vi "APDStageScan.vi"(3 "error in (no error)":errorcluster, 4 "Take Trajectory?":bool, 5 "Scanning parameters":T1) -> (0 "error out":errorcluster, 2 "output array":u32[][](array[numeric]))   [LabVIEW 2015]
uses:
  <vilib>/DAQmx/write.llb/DAQmx Write (Analog 1D Wfm NChan NSamp).vi
  <vilib>/DAQmx/write.llb/DAQmx Write (Digital Bool 1Line 1Point).vi
  <vilib>/DAQmx/read.llb/DAQmx Read (Counter 1D U32 1Chan NSamp).vi
  <vilib>/DAQmx/create/channels.llb/DAQmx Create Channel (CI-Period).vi
  <vilib>/DAQmx/configure/timing.llb/DAQmx Timing (Implicit).vi
  <vilib>/DAQmx/create/channels.llb/DAQmx Create Channel (AO-Voltage-Basic).vi
  <vilib>/DAQmx/create/channels.llb/DAQmx Create Channel (CO-Pulse Generation-Frequency).vi
  <vilib>/DAQmx/configure/timing.llb/DAQmx Timing (Sample Clock).vi
  <vilib>/DAQmx/miscellaneous.llb/DAQmx Fill In Error Info.vi
  <vilib>/DAQmx/create/channels.llb/DAQmx Create Channel (DO-Digital Output).vi
  <resource>/objmgr/daqmx.rc
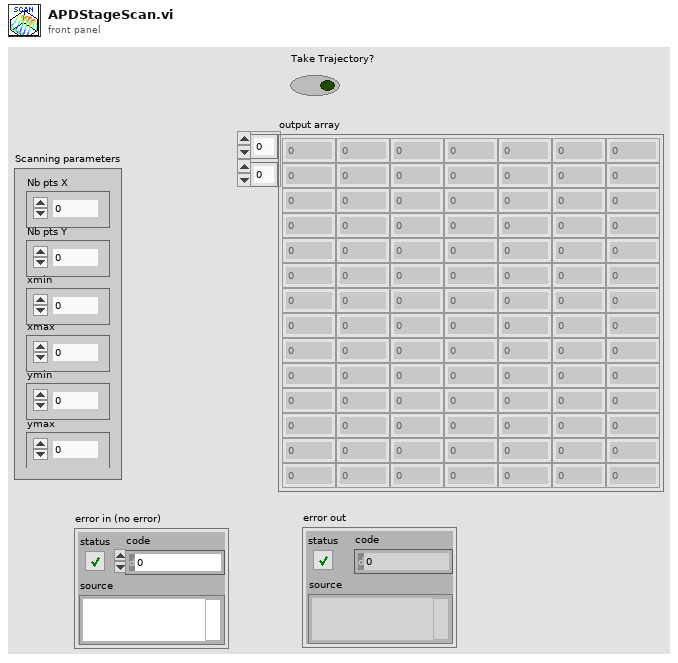
[diagram p1: front panel]
types:
  T1 = cluster{"Nb pts X":u32, "Nb pts Y":u32, "xmin":dbl, "xmax":dbl, "ymin":dbl, "ymax":dbl}
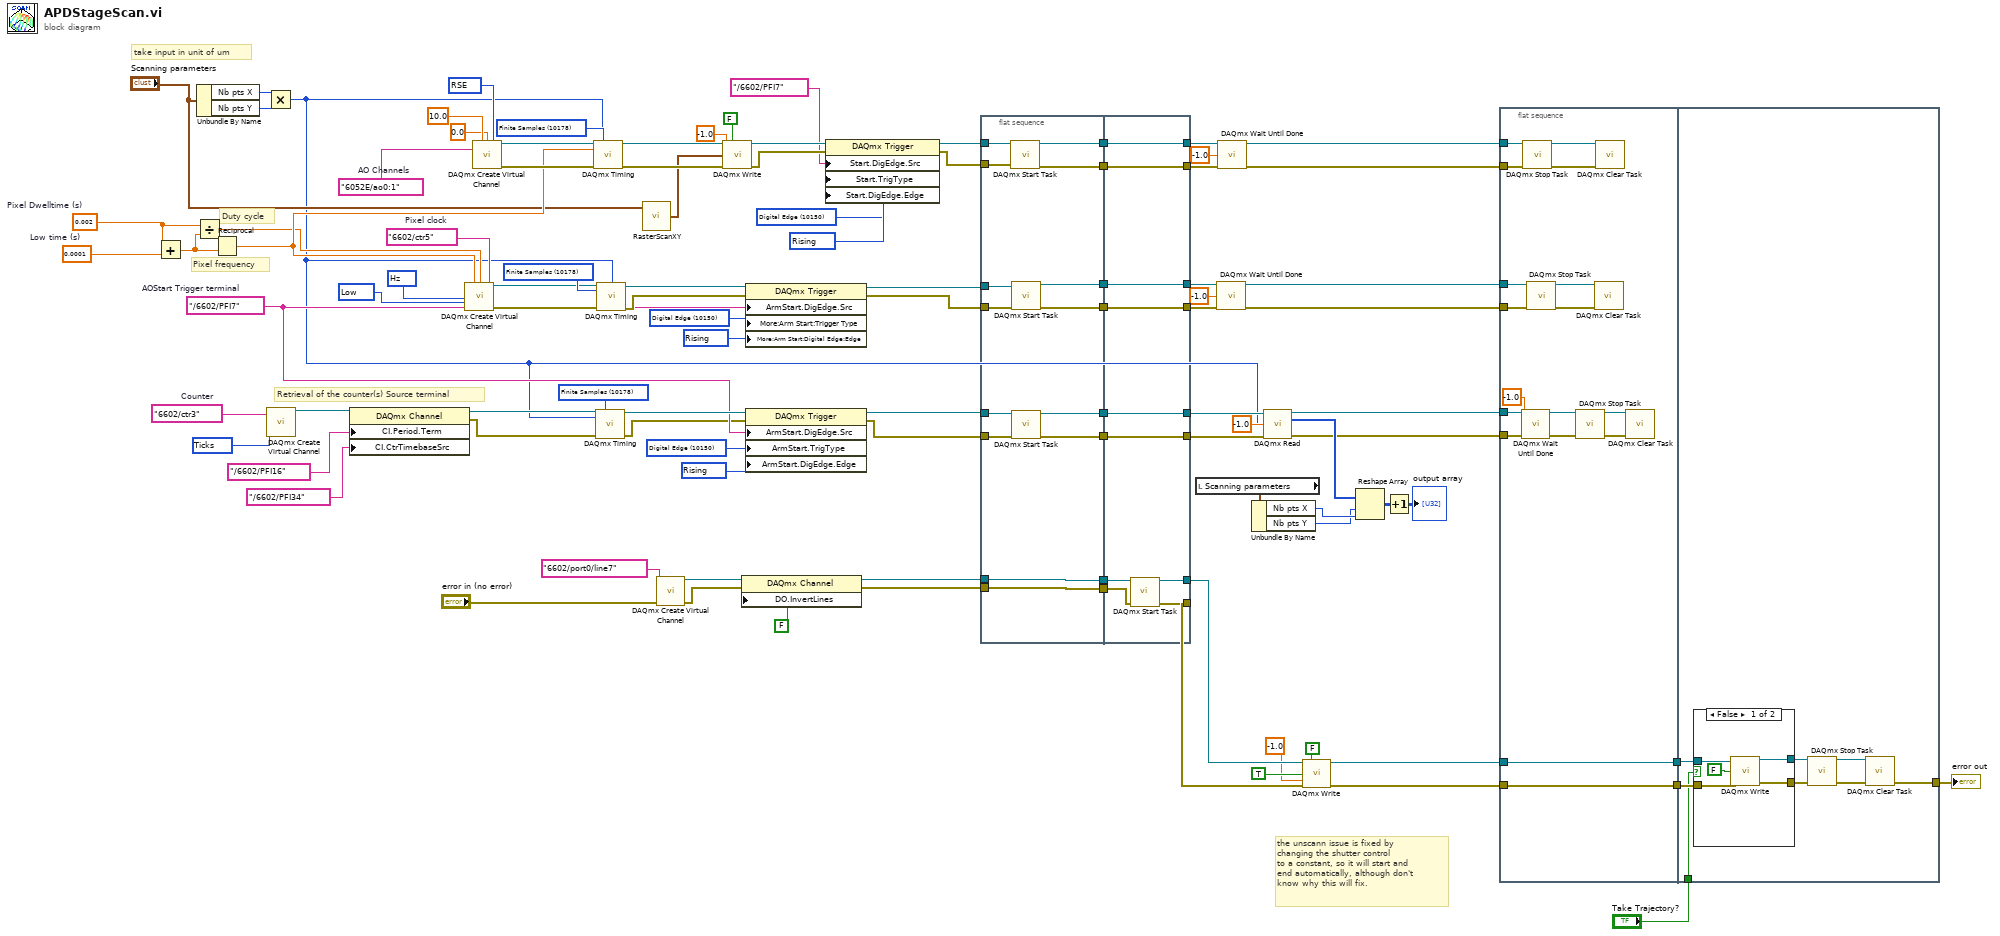
[diagram p0: block diagram]
diagram:
  w98 = 0.0001  # Low time (s)
  w95 = 0.002  # Pixel Dwelltime (s)
  w25 = 10150 items=["Analog Edge"=10099, "Digital Edge"=10150, "Digital Pattern"=10398, "Analog Window"=10103, "None"=10230] ("Start.TrigType")
  w26 = 10280 items=["Rising"=10280, "Falling"=10171] ("Start.DigEdge.Edge")
  w30 = 10083 items=["Default"=-1, "RSE"=10083, "Differential"=10106, "Pseudodifferential"=12529] ("output terminal configuration")
  w44 = 10304 items=["Seconds"=10364, "Ticks"=10304, "From Custom Scale"=10065] ("units")
  w50 = 10280 items=["Rising"=10280, "Falling"=10171] ("ArmStart.DigEdge.Edge")
  w51 = 10150 items=["Digital Edge"=10150, "None"=10230] ("ArmStart.TrigType")
  w93 = tag "6602/ctr5"  # Pixel clock
  w99 = tag "6052E/ao0:1"  # AO Channels
  w49 = tag "/6602/PFI7"  # AOStart Trigger terminal
  w84 = tag "6602/ctr3"  # Counter
  w85 = 10178 items=["Finite Samples"=10178, "Continuous Samples"=10123] ("sample mode")
  w88 = 10280 items=["Rising"=10280, "Falling"=10171] ("ArmStart.DigEdge.Edge")
  w89 = 10150 items=["Digital Edge"=10150, "None"=10230] ("ArmStart.TrigType")
  w92 = 10178 items=["Finite Samples"=10178, "Continuous Samples"=10123] ("sample mode")
  w90 = 10373 items=["Hz"=10373] ("units")
  w91 = 10214 items=["High"=10192, "Low"=10214] ("Idle State")
  w102 = 10178 items=["Finite Samples"=10178, "Continuous Samples"=10123] ("sample mode")
  # "take input in unit of um"
  # "the unscann issue is fixed by \nchanging the shutter control \nto a constant, so it will start and \nend automatically, although don't \nknow why this will fix."
  # "Retrieval of the counter(s) Source terminal"
  # "Duty cycle"
  # "Pixel frequency"
  n1 = Add(x=w95, y=w98) -> (x+y=w96:dbl)
  n2 = Divide(x=w95, y=w96) -> (x/y=w94:dbl)
  n3 = Unbundle By Name("Scanning parameters") -> ("Nb pts X"=w62:u32, "Nb pts Y"=w61:u32)
  n4 = Reciprocal(x=w96) -> (1/x=w97:dbl)
  n5 = Multiply(x=w62, y=w61) -> (x*y=w6:u32)
  n6 = call-poly <vilib>:"DAQmx Create Virtual Channel.vi"("counter"=w84, "units"=w44) -> ("task out"=w81:refnum<k21>)  [unwired: 12 in, 1 out]
  n7 = property class="DAQmx Channel"(reference=w81, "CI.Period.Term"=tag "/6602/PFI16", "CI.CtrTimebaseSrc"=tag "/6602/PFI34") -> (reference out=w80:refnum<k21>, error out=w77:errorcluster)  [unwired: 1 in]
  n8 = call-poly <vilib>:"DAQmx Create Virtual Channel.vi"("frequency"=w97, "duty cycle"=w94, "counter"=w93, "units"=w90, "idle state"=w91) -> ("task out"=w87:refnum<k21>, "error out"=w86:errorcluster)  [unwired: 9 in]
  n9 = call-poly <vilib>:"DAQmx Create Virtual Channel.vi"("maximum value"=10.0, "minimum value"=0.0, "output terminal configuration"=w30, "physical channels"=w99) -> ("task out"=w100:refnum<k21>, "error out"=w101:errorcluster)  [unwired: 10 in]
  n10 = call-poly <vilib>:"DAQmx Timing.vi"("task/channels in"=w100, "sample mode"=w102, "samples per channel"=w6, "rate"=w97, "error in"=w101) -> ("task out"=w45:refnum<k21>, "error out"=w72:errorcluster)  [unwired: 9 in]
  n11 = call-poly <vilib>:"DAQmx Timing.vi"("task/channels in"=w80, "sample mode"=w85, "samples per channel"=w6, "error in"=w77) -> ("task out"=w66:refnum<k21>, "error out"=w21:errorcluster)  [unwired: 10 in]
  n12 = call-poly <vilib>:"DAQmx Timing.vi"("task/channels in"=w87, "sample mode"=w92, "samples per channel"=w6, "error in"=w86) -> ("task out"=w83:refnum<k21>, "error out"=w82:errorcluster)  [unwired: 10 in]
  n13 = call "RasterScanXY.vi"("Scanning parameters"="Scanning parameters") -> ("X,Y AO Waveforms"=w64:waveform(dbl)[])  [unwired: 4 in]
  n14 = call-poly <vilib>:"DAQmx Create Virtual Channel.vi"("lines"=tag "6602/port0/line7", "error in"="error in (no error)") -> ("task out"=w58:refnum<k21>, "error out"=w56:errorcluster)  [unwired: 12 in]
  n15 = call-poly <vilib>:"DAQmx Write.vi"("task/channels in"=w45, "auto start"=FALSE, "data"=w64, "timeout"=-1.0, "error in"=w72) -> ("task out"=w76:refnum<k21>, "error out"=w24:errorcluster)  [unwired: 8 in, 1 out]
  n16 = property class="DAQmx Channel"(reference=w58, error in=w56, "DO.InvertLines"=FALSE) -> (reference out=w48:refnum<k21>, error out=w47:errorcluster)
  n17 = property class="DAQmx Trigger"(reference=w83, error in=w82, "ArmStart.DigEdge.Src"=w49, "More:Arm Start:Trigger Type"=w89, "More:Arm Start:Digital Edge:Edge"=w88) -> (reference out=w74:refnum<k21>, error out=w69:errorcluster)
  n18 = property class="DAQmx Trigger"(reference=w66, error in=w21, "ArmStart.DigEdge.Src"=w49, "ArmStart.TrigType"=w51, "ArmStart.DigEdge.Edge"=w50) -> (reference out=w52:refnum<k21>, error out=w20:errorcluster)
  n19 = property class="DAQmx Trigger"(reference=w76, error in=w24, "Start.DigEdge.Src"=tag "/6602/PFI7", "Start.TrigType"=w25, "Start.DigEdge.Edge"=w26) -> (reference out=w27:refnum<k21>, error out=w23:errorcluster)
  n20 = flat-sequence {
    tunnel: w27 -> [w116]
    tunnel: w74 -> [w115]
    tunnel: w23 -> [w104]
    tunnel: w69 -> [w106]
    tunnel: w20 -> [w110]
    tunnel: w52 -> [w109]
    tunnel: w48 -> [w108]
    tunnel: w47 -> [w107]
    tunnel: [w105] -> w42
    tunnel: [w114] -> w41
    tunnel: [w103] -> w40
    tunnel: [w113] -> w39
    tunnel: [w112] -> w38
    tunnel: [w111] -> w37
    tunnel: [w108] -> w36
    tunnel: [w107] -> w35
    tunnel: [w120] -> w46
    tunnel: [w122] -> w68
    tunnel: [w123] -> w15
    tunnel: [w124] -> w32
    tunnel: [w119] -> w71
    tunnel: [w125] -> w73
    tunnel: [w126] -> w43
    tunnel: w42 -> [w126]
    tunnel: w41 -> [w125]
    tunnel: w40 -> [w119]
    tunnel: w39 -> [w124]
    tunnel: w38 -> [w123]
    tunnel: w37 -> [w122]
    tunnel: w36 -> [w121]
    tunnel: w35 -> [w118]
    tunnel: [w117] -> w34
    frame #0 {
      n21 = call <vilib>:"DAQmx Start Task.vi"("task/channels in"=w116, "error in"=w104) -> ("task out"=w105:refnum<k21>, "error out"=w103:errorcluster)  [unwired: 12 in]
      n22 = call <vilib>:"DAQmx Start Task.vi"("task/channels in"=w115, "error in"=w106) -> ("task out"=w114:refnum<k21>, "error out"=w113:errorcluster)  [unwired: 12 in]
      n23 = call <vilib>:"DAQmx Start Task.vi"("task/channels in"=w109, "error in"=w110) -> ("task out"=w111:refnum<k21>, "error out"=w112:errorcluster)  [unwired: 12 in]
    }
    frame #1 {
      n24 = call <vilib>:"DAQmx Start Task.vi"("task/channels in"=w121, "error in"=w118) -> ("task out"=w120:refnum<k21>, "error out"=w117:errorcluster)  [unwired: 12 in]
    }
  }
  n25 = local read "Scanning parameters"() -> (w60:T1)
  n26 = call <vilib>:"DAQmx Wait Until Done.vi"("task/channels in"=w73, "timeout (sec)"=-1.0, "error in"=w32) -> ("task out"=w33:refnum<k21>, "error out"=w31:errorcluster)  [unwired: 11 in]
  n27 = call <vilib>:"DAQmx Wait Until Done.vi"("task/channels in"=w43, "timeout (sec)"=-1.0, "error in"=w71) -> ("task out"=w75:refnum<k21>, "error out"=w70:errorcluster)  [unwired: 11 in]
  n28 = Unbundle By Name(w60) -> ("Nb pts X"=w17:u32, "Nb pts Y"=w16:u32)
  n29 = call-poly <vilib>:"DAQmx Read.vi"("task/channels in"=w68, "number of samples per channel"=w6, "timeout"=-1.0, "error in"=w15) -> ("task out"=w67:refnum<k21>, "data"=w59:u32[], "error out"=w14:errorcluster)  [unwired: 9 in]
  n30 = call-poly <vilib>:"DAQmx Write.vi"("task/channels in"=w46, "auto start"=FALSE, "data"=TRUE ("Start"), "timeout"=-1.0, "error in"=w34) -> ("task out"=w11:refnum<k21>, "error out"=w9:errorcluster)  [unwired: 8 in, 1 out]
  n31 = Reshape Array(w59, w16, w17) -> (w5:u32[][])
  n32 = Increment(x=w5) -> (x+1=→"output array":u32[][])
  n33 = flat-sequence {
    tunnel: w75 -> [w143]
    tunnel: w70 -> [w140]
    tunnel: w67 -> [w133]
    tunnel: w33 -> [w132]
    tunnel: w31 -> [w131]
    tunnel: w14 -> [w129]
    tunnel: w11 -> [w128]
    tunnel: [w128] -> w10
    tunnel: w9 -> [w127]
    tunnel: [w127] -> w8
    tunnel: w10 -> [w148]
    tunnel: w8 -> [w146]
    tunnel: [w149] -> w3
    tunnel: "Take Trajectory?" -> [w144]
    frame #0 {
      n34 = call <vilib>:"DAQmx Wait Until Done.vi"("task/channels in"=w133, "timeout (sec)"=-1.0, "error in"=w129) -> ("task out"=w134:refnum<k21>, "error out"=w136:errorcluster)  [unwired: 11 in]
      n35 = call <vilib>:"DAQmx Stop Task.vi"("task/channels in"=w143, "error in"=w140) -> ("task out"=w142:refnum<k21>, "error out"=w139:errorcluster)  [unwired: 12 in]
      n36 = call <vilib>:"DAQmx Stop Task.vi"("task/channels in"=w132, "error in"=w131) -> ("task out"=w141:refnum<k21>, "error out"=w138:errorcluster)  [unwired: 12 in]
      n37 = call <vilib>:"DAQmx Stop Task.vi"("task/channels in"=w134, "error in"=w136) -> ("task out"=w135:refnum<k21>, "error out"=w137:errorcluster)  [unwired: 12 in]
      n38 = call <vilib>:"DAQmx Clear Task.vi"("task in"=w141, "error in"=w138) -> ()  [unwired: 13 in, 1 out]
      n39 = call <vilib>:"DAQmx Clear Task.vi"("task in"=w142, "error in"=w139) -> ()  [unwired: 13 in, 1 out]
      n40 = call <vilib>:"DAQmx Clear Task.vi"("task in"=w135, "error in"=w137) -> ()  [unwired: 13 in, 1 out]
    }
    frame #1 {
      n41 = case shown="False" w144 {
        tunnel: w148 -> [w156 w157]
        tunnel: [w155 w157] -> w147
        tunnel: w146 -> [w154 w158]
        tunnel: [w153 w158] -> w145
        frame False {
          n42 = call-poly <vilib>:"DAQmx Write.vi"("task/channels in"=w156, "data"=FALSE, "error in"=w154) -> ("task out"=w155:refnum<k21>, "error out"=w153:errorcluster)  [unwired: 10 in, 1 out]
        }
        frame True {
        }
      }
      n43 = call <vilib>:"DAQmx Stop Task.vi"("task/channels in"=w147, "error in"=w145) -> ("task out"=w150:refnum<k21>, "error out"=w151:errorcluster)  [unwired: 12 in]
      n44 = call <vilib>:"DAQmx Clear Task.vi"("task in"=w150, "error in"=w151) -> ("error out"=w149:errorcluster)  [unwired: 13 in]
    }
  }
  "error out" <- w3
